vi "StringSubSet (SubVI).vi"(8 "Удалить кавычки":bool, 11 "<JSON> in":string) -> (3 "<JSON> out":string)   [LabVIEW 2017, in "LV_Unicorn.lvlib"]
uses:
  LV_Unicorn.lvlib
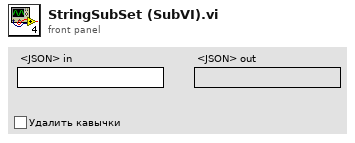
[diagram p1: front panel]
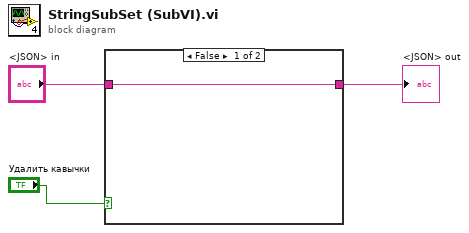
[diagram p0: block diagram]
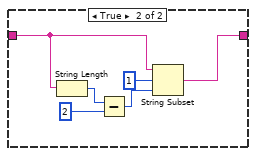
[diagram p2: hidden frame]
diagram:
  n1 = case shown="False" "Удалить кавычки" {
    tunnel: [w4 w10] -> w3
    tunnel: "<JSON> in" -> [w4 w9]
    frame False {
    }
    frame True {
      n2 = String Length(string=w9) -> (length=w6:i32)
      n3 = Subtract(x=w6, y=2) -> (x-y=w5:i32)
      n4 = String Subset(string=w9, offset (0)=1, length (rest)=w5) -> (substring=w10:string)
    }
  }
  "<JSON> out" <- w3
